vi "Test_LogIfError_IncomingError_ErrorLogged.vi"(8 "error in (no error)":errorcluster, 11 "TestCase in":refnum<class "TestComposedLog.lvclass">) -> (0 "error out":errorcluster, 3 "TestCase out":refnum<class "TestComposedLog.lvclass">)   [LabVIEW 2017, in "TestComposedLog.lvclass"]
uses:
  TestComposedLog.lvclass
  Source/Composed Log/Types/Log Level.ctl
  Source/Composed Log/LoggerReference/LoggerReference.lvclass/LoggerReference.ctl
  Source/LVQueue Sink/LVQueue Sink.lvclass/LVQueue Sink.ctl
  37526c0e-e1d4-486f-9419-58d832469ea5.vi
  37526c0e-e1d4-486f-9419-58d832469ea5.vi/72fe5bdf-3db3-4ec4-aaed-8915ffd3ee65.vi
  Source/Composed Log/LoggerReference/Return Aggregate Queues.vi
  Source/Composed Log/LoggerReference/Add Aggregate Log.vi
  37526c0e-e1d4-486f-9419-58d832469ea5.vi/72fe5bdf-3db3-4ec4-aaed-8915ffd3ee65.vi/a64c4407-b312-4eef-9b09-3934c689987f.vi
  Source/Composed Log/LoggerReference/Send Add Sink.vi
  Source/LVQueue Sink/LVQueue Sink.lvclass
  C:/CS/Internal/LabVIEW/Logger/Source/Composed Log/Log Sink/Log Sink.lvclass
  Source/Composed Log/Application Logger/Launch Worker Loop.vi
  Source/Composed Log/LoggerReference/Initialize Logger Instance.vi
  Source/Composed Log/Singleton Event Log/Logger Queue FGV.vi
  Source/Composed Log/IErrorFormat/IErrorFormat.lvclass
  Source/Composed Log/LoggerReference/LoggerReference.lvclass
  Source/Composed Log/Log Sink/Log Sink.lvclass
  <vilib>/addons/_JKI Toolkits/VI Tester/TestCase.llb/TestCase.lvclass
  Source/Composed Log/Singleton Event Log/Singleton Event Log.lvlib
  Source/Composed Log/Composed Log.lvlib
  C:/Program Files (x86)/National Instruments/LabVIEW 2017/vi.lib/addons/_JKI Toolkits/VI Tester/TestCase.llb/TestCase.lvclass
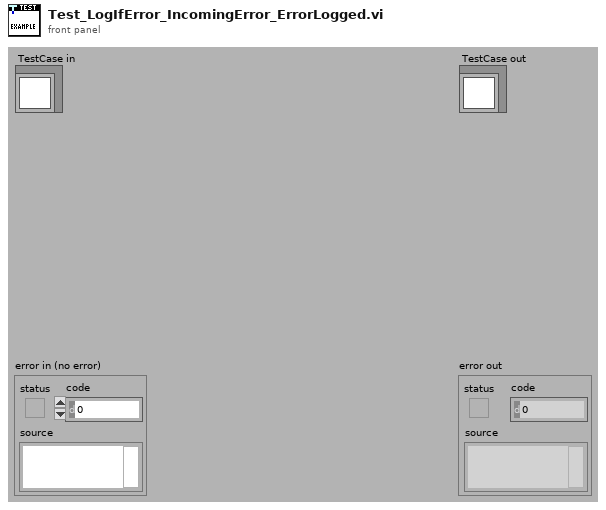
[diagram p1: front panel]
types:
  T1 = typedef "Composed Log.lvlib/Log Level.ctl" = enum16{"Debug", "Info", "Warning", "Error", "Critical"}
  T2 = typedef "Composed Log.lvlib/Log Packet.ctl" = cluster{"Data To Log":string, "Source":string, "Event Level":T1, "Event Time":timestamp}
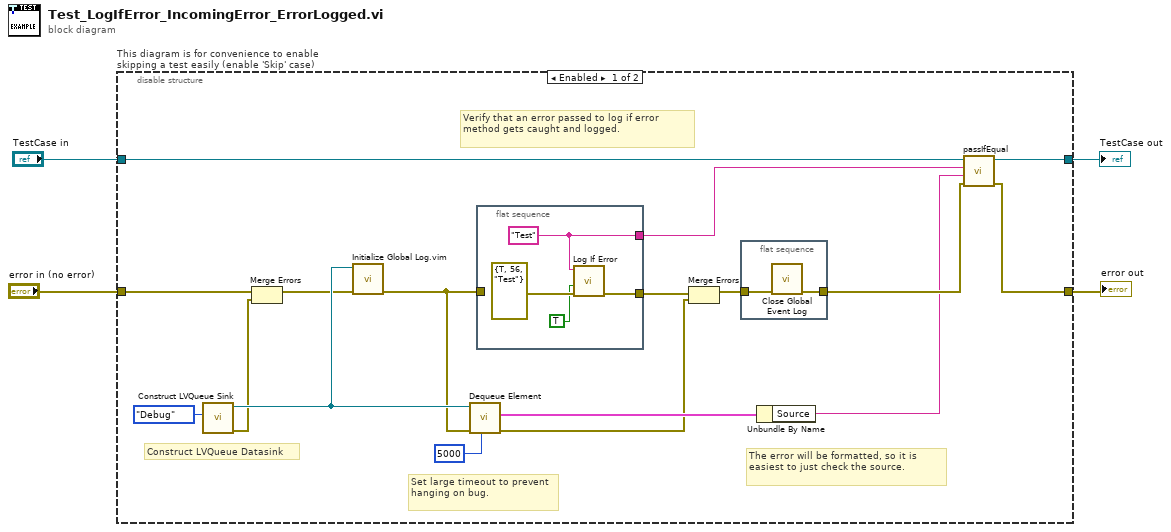
[diagram p0: block diagram]
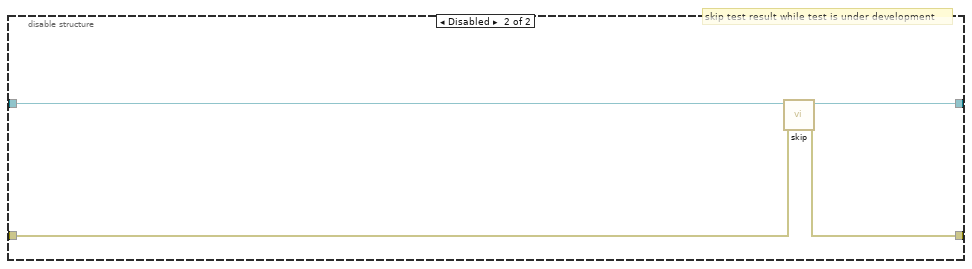
[diagram p2: hidden frame]
diagram:
  n1 = disable-structure "This diagram is for convenience to enable skipping a test easily (enable 'Skip' case)" shown="Enabled" {
    disable-tunnel: "TestCase in" -> [w9 w31]
    disable-tunnel: [w8 w29] -> w1
    disable-tunnel: [w10 w30] -> w3
    disable-tunnel: "error in (no error)" -> [w21 w28]
    frame Enabled {
      # "The error will be formatted, so it is easiest to just check the source."
      # "Construct LVQueue Datasink"
      # "Set large timeout to prevent hanging on bug."
      # "Verify that an error passed to log if error method gets caught and logged."
      n2 = call "Construct LVQueue Sink.vi"("LogLevel"=Log_Level."Debug") -> ("error out"=w15:errorcluster, "LVQueue Sink out"=w19:refnum<class "LVQueue Sink.lvclass">)  [unwired: 9 in]
      n3 = Merge Errors(w21, w15) -> (w16:errorcluster)
      n4 = call "Initialize Global Log.vim"("error in (no error)"=w16, "Log Sink(s)"=w19) -> ("error out"=w14:errorcluster)  [unwired: 8 in, 1 out]
      n5 = call "Dequeue Element.vi"("timeout in ms (-1)"=5000, "error in (no error)"=w14, "LVQueue Sink in"=w19) -> ("error out"=w13:errorcluster, "Log Packet"=w17:T2)  [unwired: 5 in, 2 out]
      n6 = flat-sequence {
        tunnel: w14 -> [_]
        tunnel: [w24] -> w6
        tunnel: [w23] -> w5
        frame #0 {
          w24 = "Test" ("SourceID")
          n7 = call "Log If Error.vi"("Error In"=errorcluster {"status"=TRUE, "code"=56, "source"="Test"}, "Clear After Logging?(F)"=TRUE ("Clear Error?(F)"), "SourceID"=w24) -> ("error out"=w23:errorcluster)  [unwired: 8 in]
        }
      }
      n8 = Merge Errors(w5, w13) -> (w12:errorcluster)
      n9 = flat-sequence {
        tunnel: [w27] -> w11
        tunnel: w12 -> [w26]
        frame #0 {
          n10 = call "Close Global Event Log.vi"("error in (no error)"=w26) -> ("error out"=w27:errorcluster)  [unwired: 10 in]
        }
      }
      n11 = Unbundle By Name(w17) -> ("Source"=w7:string)
      n12 = call-dynamic "passIfEqual.vi"("error in (no error)"=w11, "y"=w7, "x"=w6, "TestCase in"=w9) -> ("error out"=w10:errorcluster, "TestCase out"=w8:refnum<class "TestComposedLog.lvclass">)  [unwired: 6 in]
    }
    frame Disabled {
      # "skip test result while test is under development"
      n13 = call <vilib>:"skip.vi"("error in (no error)"=w28, "TestCase in"=w31) -> ("error out"=w30:errorcluster, "TestCase out"=w29:refnum<class "TestComposedLog.lvclass">)  [unwired: 8 in]
    }
  }
  "error out" <- w3
  "TestCase out" <- w1
